vi "cameraStop.vi"(8 "error in (no error)":errorcluster, 11 "WinX32Camera in":refnum<class "WinX32Camera.lvclass">) -> (0 "error out":errorcluster, 3 "WinX32Camera out":refnum<class "WinX32Camera.lvclass">)   [LabVIEW 2011, in "WinX32Camera.lvclass"]
uses:
  WinX32Camera.lvclass
  WinX32Camera.lvclass/WinX32Camera.ctl
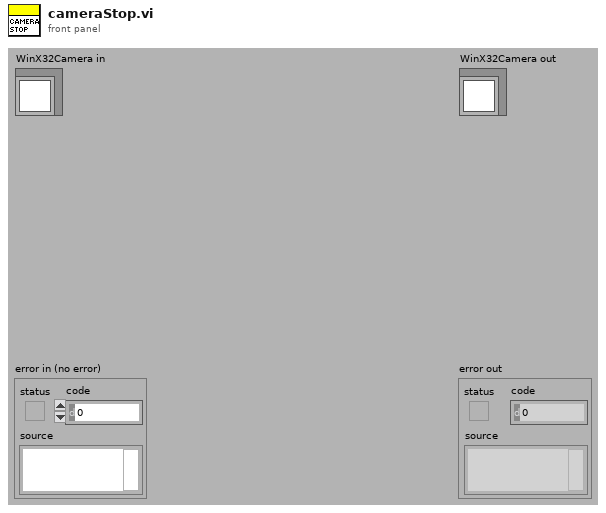
[diagram p1: front panel]
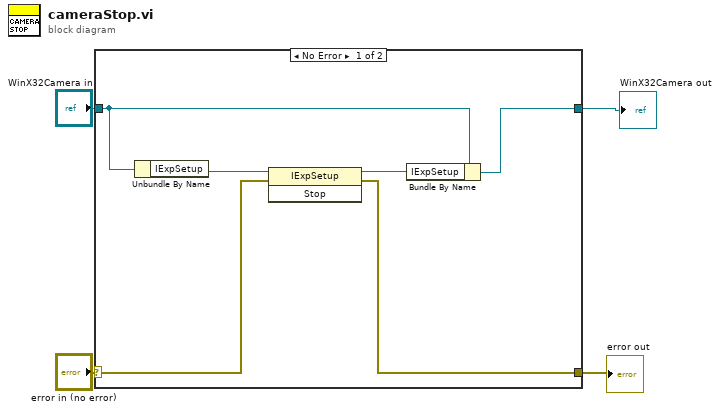
[diagram p0: block diagram]
diagram:
  n1 = case shown="No Error" "error in (no error)" {
    selector: "error in (no error)" -> [w6 w12]
    tunnel: [w5 w12] -> w3
    tunnel: [w10 w11] -> w1
    tunnel: "WinX32Camera in" -> [w9 w11]
    frame No Error {
      n2 = Unbundle By Name(w9) -> ("IExpSetup"=w8:refnum<k7>)
      n3 = invoke class="IExpSetup" method="Stop"(reference=w8, error in=w6) -> (reference out=w7:refnum<k7>, error out=w5:errorcluster)  [unwired: 1 in, 1 out]
      n4 = Bundle By Name(cluster=w9, "IExpSetup"=w7) -> (w10:refnum<class "WinX32Camera.lvclass">)
    }
    frame Error {
    }
  }
  "error out" <- w3
  "WinX32Camera out" <- w1
